vi "Error To String.vi"(11 "error in (no error)":errorcluster) -> (3 "String":string)   [LabVIEW 2020, in "RTAF.lvlib" / "Alarms Handler Actor.lvclass"]
uses:
  Alarms Handler Actor.lvclass
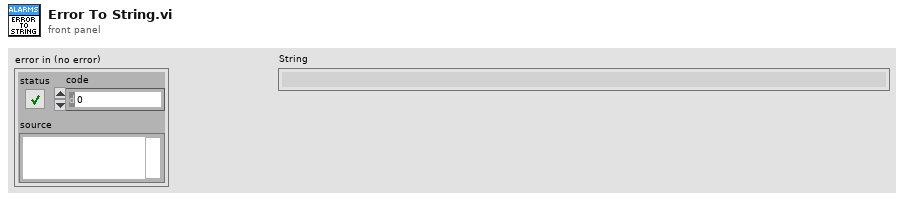
[diagram p1: front panel]
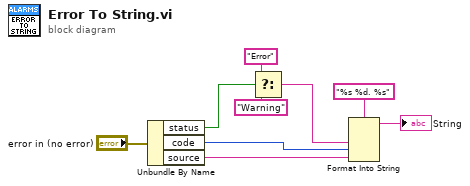
[diagram p0: block diagram]
diagram:
  n1 = Unbundle By Name("error in (no error)") -> ("status"=w4:bool, "code"=w5:i32, "source"=w8:string)
  n2 = Select(t="Error", s=w4, f="Warning") -> (s? t:f=w1:string)
  n3 = Format Into String(format string="%s %d. %s", w1, w5, w8) -> (resulting string=→"String":string)  [unwired: 2 in, 1 out]
